vi "Wait for Aqusition duration.vi"(8 "error in (no error)":errorcluster, 10 "Aqusition Time (s)":dbl, 11 "DAQ Process in":refnum<class "DAQ Process.lvclass">) -> (0 "error out":errorcluster, 3 "DAQ Process\\":refnum<class "DAQ Process.lvclass">)   [LabVIEW 2022 SP3, in "DAQ Process.lvlib" / "DAQ Process.lvclass"]
uses:
  DAQ Process.lvclass
  DAQ Process.lvclass/DAQ Process.ctl
  XY Stage/Process Actor/Process Framework/Process State Data/Process State Data.lvclass
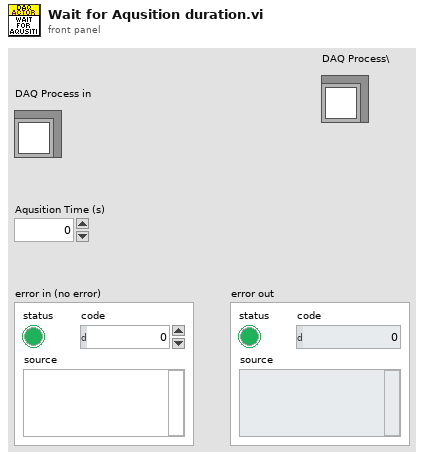
[diagram p1: front panel]
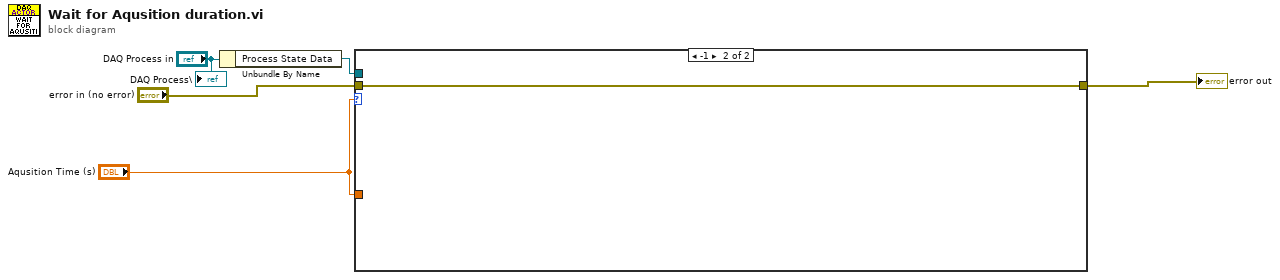
[diagram p0: block diagram]
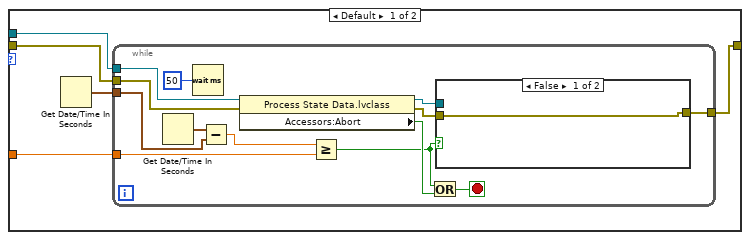
[diagram p2: hidden frame]
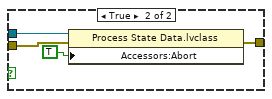
[diagram p3: hidden frame]
diagram:
  n1 = Unbundle By Name("DAQ Process in") -> ("Process State Data"=w3:refnum<data-value>)
  n2 = case shown="-1" "Aqusition Time (s)" {
    tunnel: "Aqusition Time (s)" -> [w9 _]
    tunnel: w3 -> [w8 _]
    tunnel: "error in (no error)" -> [w7 w29]
    tunnel: [w6 w29] -> w5
    frame Default {
      n3 = Get Date/Time In Seconds() -> (seconds since 1Jan1904=w10:timestamp)
      n4 = while {
        tunnel: w10 -> [w22]
        tunnel: w9 -> [w20]
        tunnel: w8 -> [w19]
        tunnel: w7 -> [w13]
        tunnel: [w11] -> w6
        stop <- w16 stop-if-true
        n5 = Get Date/Time In Seconds() -> (seconds since 1Jan1904=w23:timestamp)
        n6 = Wait (ms)(milliseconds to wait=u32 50) -> ()  [unwired: 1 out]
        n7 = Subtract(x=w23, y=w22) -> (x-y=w21:dbl)
        n8 = property class="Process State Data.lvclass"(reference=w19, error in=w13) -> (reference out=w15:refnum<data-value>, error out=w12:errorcluster, "Accessors:Abort"=w18:bool)
        n9 = Greater Or Equal?(x=w21, y=w20) -> (x >= y?=w17:bool)
        n10 = Or(x=w17, y=w18) -> (x .or. y?=w16:bool)
        n11 = case shown="False" w17 {
          tunnel: w15 -> [_ w28]
          tunnel: w12 -> [w24 w26]
          tunnel: [w24 w25] -> w11
          frame False {
          }
          frame True {
            n12 = property class="Process State Data.lvclass"(reference=w28, error in=w26, "Accessors:Abort"=TRUE ("Abort")) -> (error out=w25:errorcluster)  [unwired: 1 out]
          }
        }
      }
    }
    frame -1 {
    }
  }
  "error out" <- w5
  "DAQ Process\\" <- "DAQ Process in"
